vi "PowerX.vi"(8 "Multiplier":dbl, 9 "Divider":dbl, 10 "Power":dbl, 11 "Signal In":dbl[](array[numeric])) -> (3 "Signal Out":dbl[](array[numeric]))   [LabVIEW 2023]
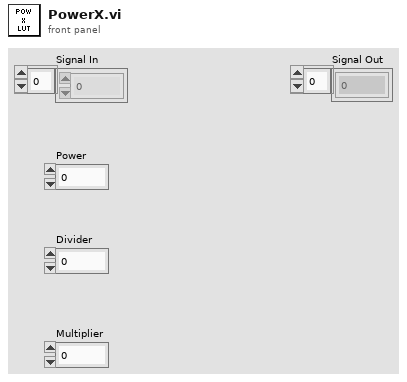
[diagram p1: front panel]
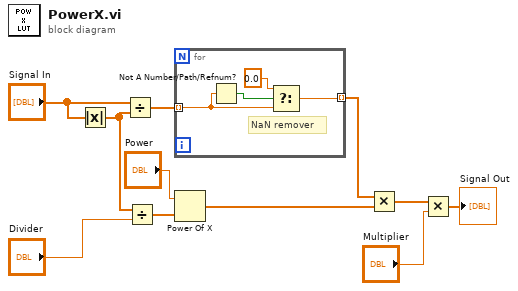
[diagram p0: block diagram]
diagram:
  n1 = Absolute Value(x="Signal In") -> (abs(x)=w1:dbl[])
  n2 = Divide(x="Signal In", y=w1) -> (x/y=w3:dbl[])
  n3 = Divide(x=w1, y="Divider") -> (x/y=w5:dbl[])
  n4 = for {
    tunnel: w3 -> [w13] mode=indexing
    tunnel: [w14] -> w4 mode=indexing
    # "NaN remover"
    n5 = Not A Number/Path/Refnum?(number/path/refnum=w13) -> (NaN/Path/Refnum?=w12:bool)
    n6 = Select(t=0.0, s=w12, f=w13) -> (s? t:f=w14:dbl)
  }
  n7 = Power Of X(1:w5, 2:"Power") -> (0:w6:dbl[])
  n8 = Multiply(x=w4, y=w6) -> (x*y=w2:dbl[])
  n9 = Multiply(x=w2, y="Multiplier") -> (x*y=→"Signal Out":dbl[])
